vi "Main.vi"() -> ()   [LabVIEW 2017]
uses:
  <vilib>/Instr/_visa.llb/VISA Configure Serial Port (Instr).vi
panel:
  in  "Select Device":u16(ring) items=["COM5 (Arduino Uno)"]
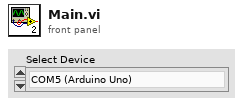
[diagram p1: front panel]
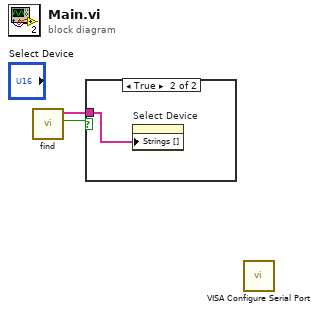
[diagram p0: block diagram]
diagram:
  n1 = call "find.vi"() -> ("have devices"=w2:bool, "find list"=w1:string[])  [unwired: 9 in, 1 out]
  n2 = case shown="True" w2 {
    tunnel: w1 -> [_ w3]
    frame False {
    }
    frame True {
      n3 = property on="Select Device" class="Ring (strict)"("Strings []"=w3) -> ()  [unwired: 2 in, 2 out]
    }
  }
  n4 = call-poly "VISA Configure Serial Port"() -> ()  [unwired: 14 in, 2 out]
